vi "HmiScheduler.vi"(7 "Param Screen Title":string, 8 "error in (no error)":errorcluster, 11 "Param Initial VI Path":path) -> (0 "error out":errorcluster)   [LabVIEW 2013]
uses:
  Ctrls/BoutonAPropos.ctl
  Ctrls/BoutonHelp.ctl
  HmiSchedulerAppConfig.ctl
  030 - EVENTS/03 - ToMessageHandlerProcess/ToMessageHandlerEvent.ctl
  030 - EVENTS/03 - ToMessageHandlerProcess/enumMessageCriticity.ctl
  050 - CONFIG/00 - ApplicationConfig/Ctrls/EnumFgvConfigCommand.ctl
  SubVis/enumDeferPanelUpdate.ctl
  030 - EVENTS/EnumFgvEventCommand.ctl
  090 - ERRORS/Ctrls/enumLogAndView.ctl
  040 - SCREENS/enumScreen.ctl
panel:
  out "Logo 600 X 200":picture
  out "ApplicationName":string
  out "ScreenTitle":string
  in  "Simulation":string
  in  "ClearError":bool
  in  "ViewError":bool
  out "LastMessage":string
  out "ProgressBar":u8(slide) scale=0.0..100.0
  out "DateTime":string
  in  "BoutonHelp":T1
  in  "BoutonAPropos":T2
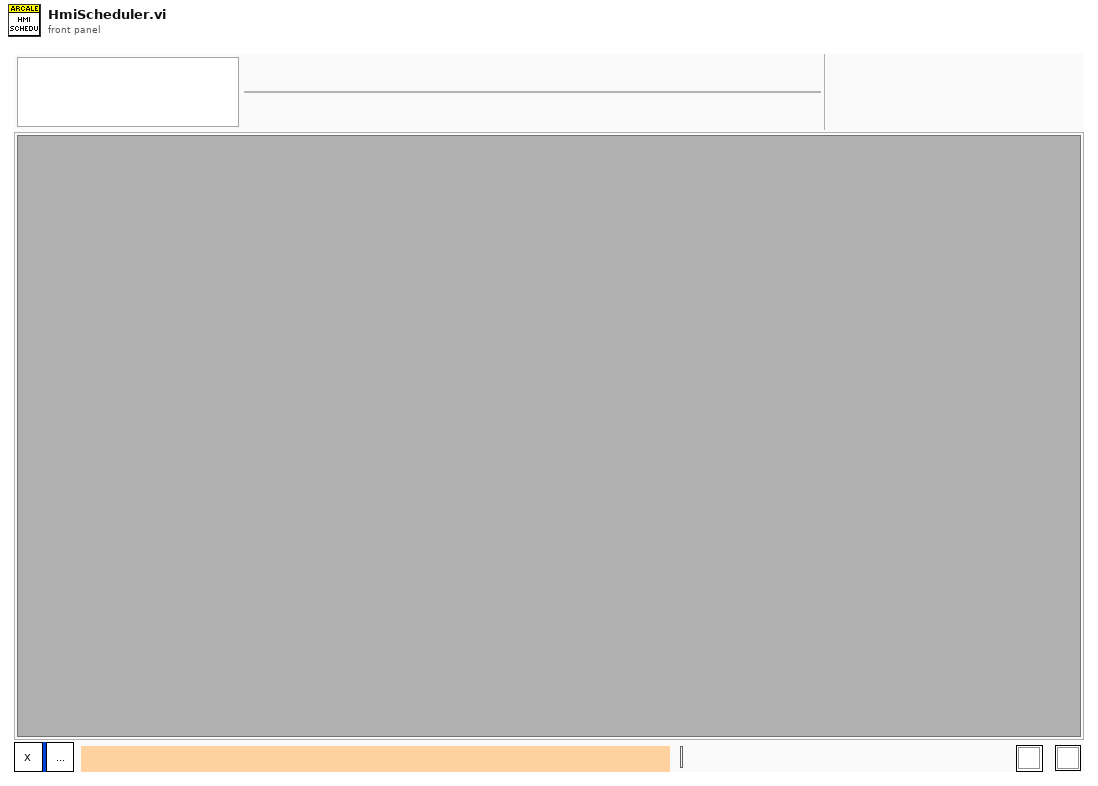
[diagram p1: front panel]
types:
  T1 = typedef "BoutonHelp.ctl" = bool
  T2 = typedef "BoutonAPropos.ctl" = bool
  T3 = typedef "HmiSchedulerAppConfig.ctl" = cluster{"Loaded VI Ref":refnum<vi>, "Loaded Vi Path":path, "AutomaticProgressBarOn":bool, "LastMessage":T4, "Previous loaded VI paths":path[], "Previous loaded Screen title":string[], "Loaded Screen title":string}
  T4 = typedef "ToMessageHandlerEvent.ctl" = cluster{"date / time":timestamp, "Criticity":T5, "Emitter":string, "Message":string}
  T5 = typedef "enumMessageCriticity.ctl" = enum16{"No error", "Info", "Warning", "Error", "Fatal error"}
  T6 = typedef "EnumFgvConfigCommand.ctl" = enum16{"Load", "Get", "Set", "Save To Disk"}
  T7 = enum32{"Invalid", "Standard", "Closed", "Hidden", "Minimized", "Maximized"}
  T8 = typedef "enumDeferPanelUpdate.ctl" = enum16{"suspend layout", "resume layout"}
  T9 = enum8{"Enabled", "Disabled", "Disabled and Grayed Out"}
  T10 = typedef "ApplicationInfos.ctl" = cluster{"ApplicationName":string, "ApplicationVersion":string, "Logo 600X200 path":path, "Logo 400X400 path":path, "Client":string}
  T11 = typedef "ApplicationConfig.ctl" = cluster{"Data Path":path, "MessageHandlerConfig":T12, "Simulation":bool, "Dictionnary":string}
  T12 = typedef "MessageHandlerConfig.ctl" = cluster{"Max log files":u32, "Max messages per file":u32}
  T13 = typedef "EnumFgvEventCommand.ctl" = enum16{"Setup", "Cleanup", "Get"}
  T14 = typedef "enumLogAndView.ctl" = enum16{"Log only", "Log and view"}
  T15 = typedef "enumScreen.ctl" = enum16{"Test screen", "Ecran principal", "LOG", "Setup", "Popup : About", "Popup : View last message", "Popup : WebBrowser help", "Traduction", "Popup : DEBUG Process"}
  T16 = typedef "ToHmiSchedulerCommand.ctl" = enum16{"Load screen", "Lock screen", "Unlock screen", "Close enable", "Close disable", "Start automatic progress bar", "Stop automatic progress bar", "Set progress bar value (0..100)", "Load previous screen", "Close application", "View message", "Clear message", "Set Window State"}
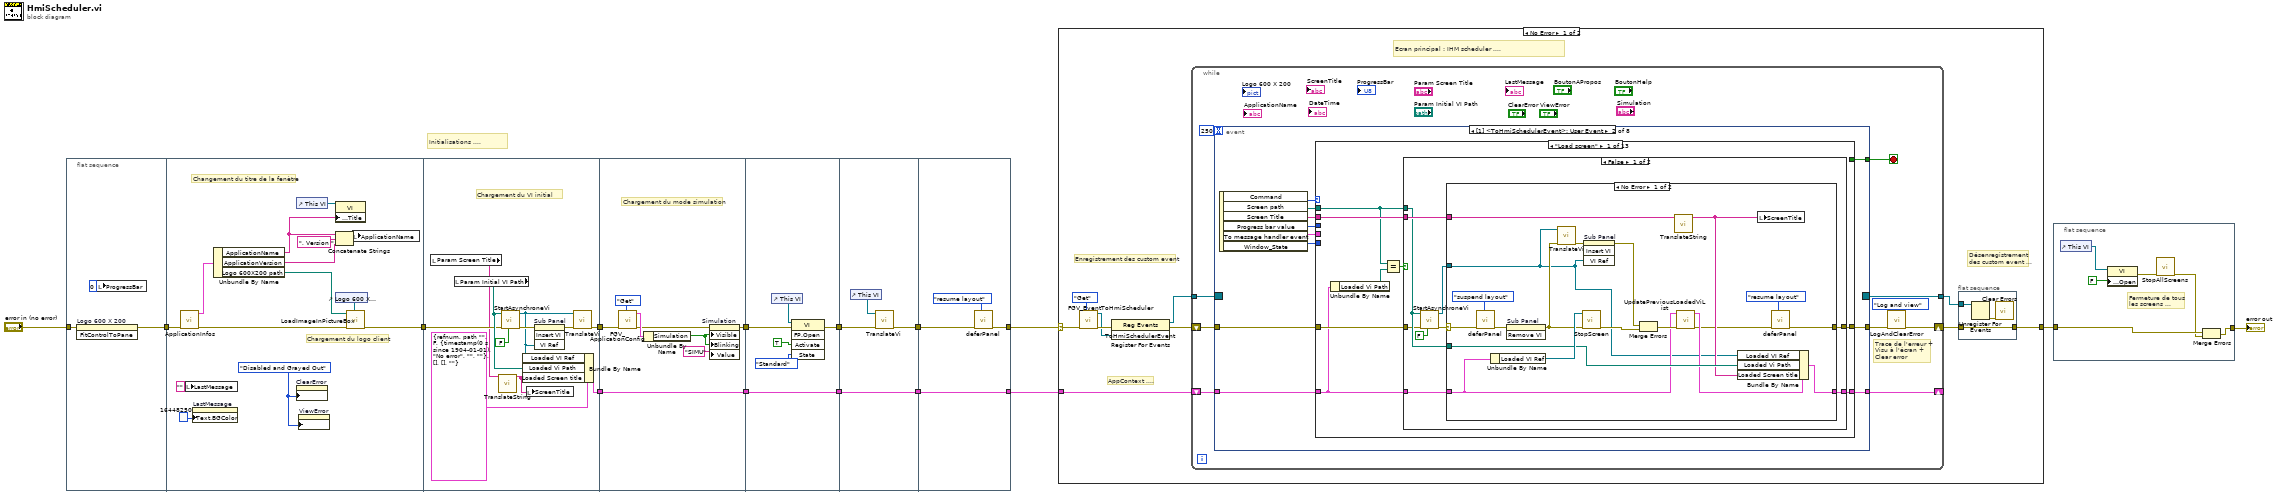
[diagram p0: block diagram]
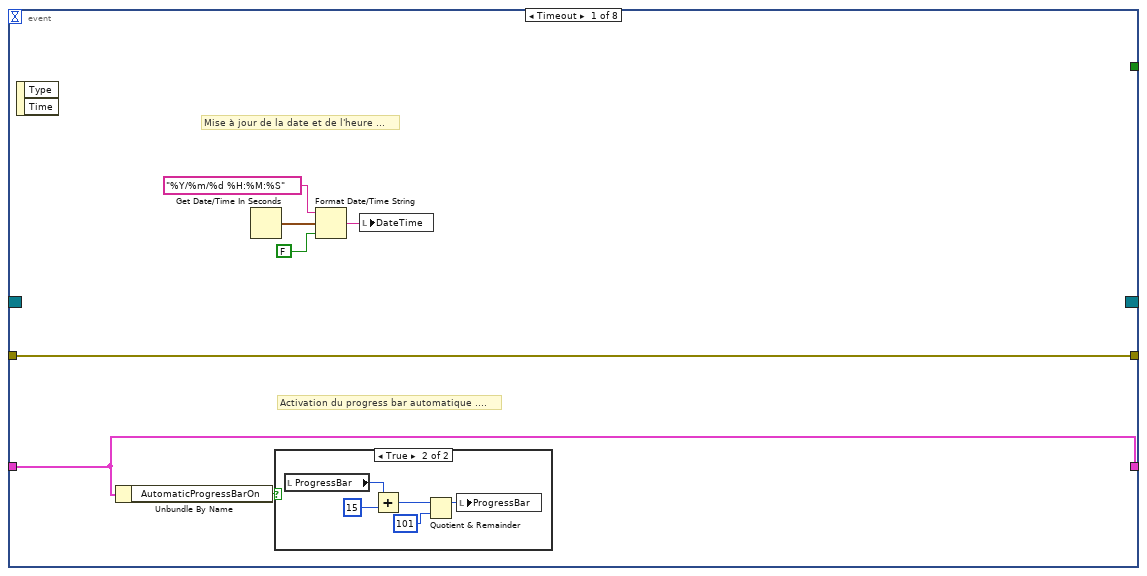
[diagram p2: hidden frame]
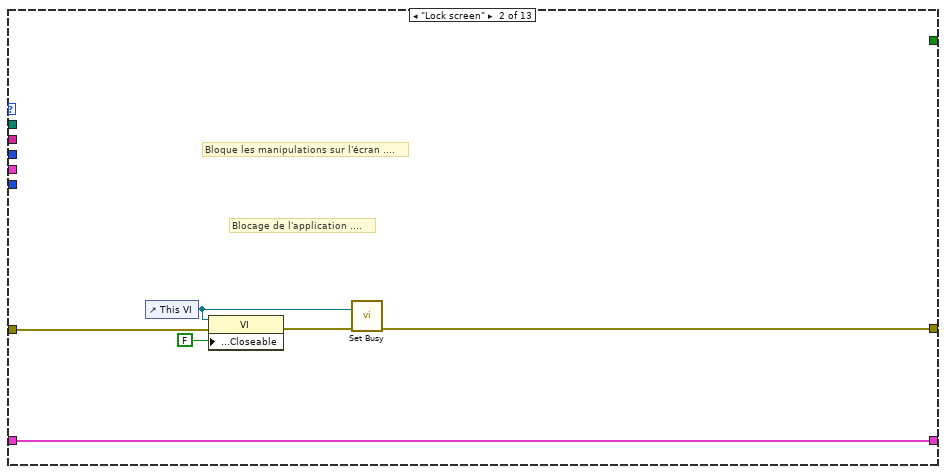
[diagram p6: hidden frame]
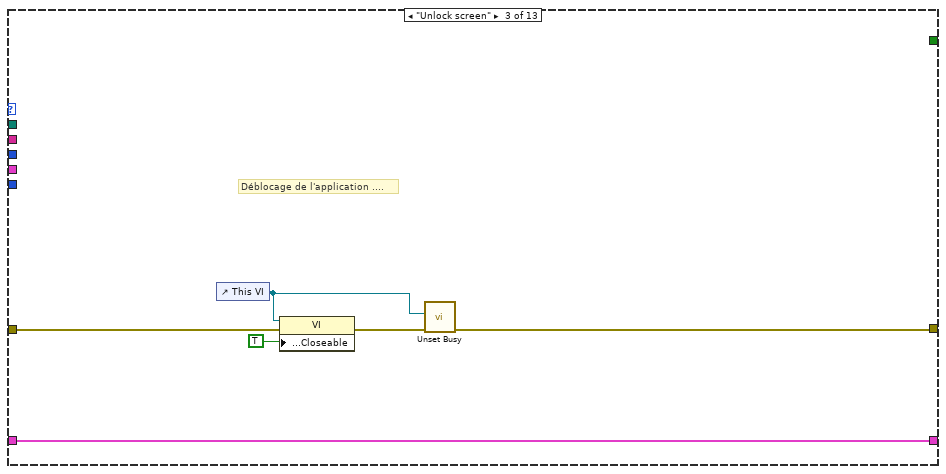
[diagram p7: hidden frame]
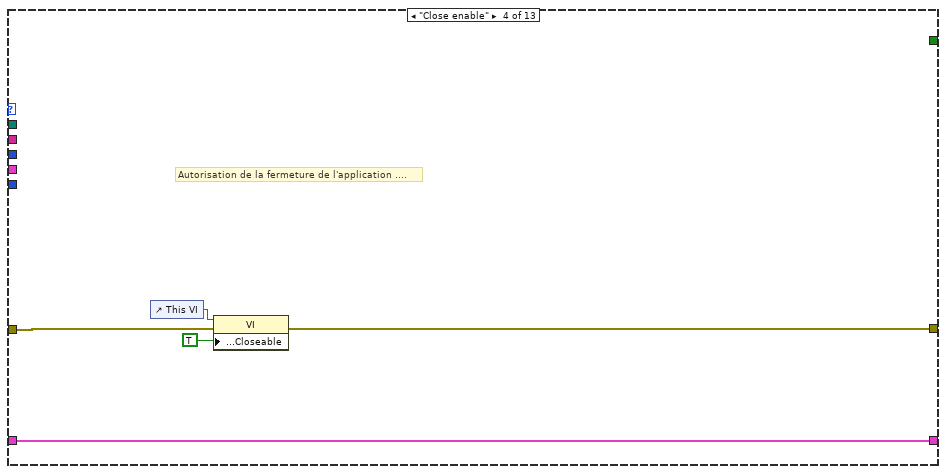
[diagram p8: hidden frame]
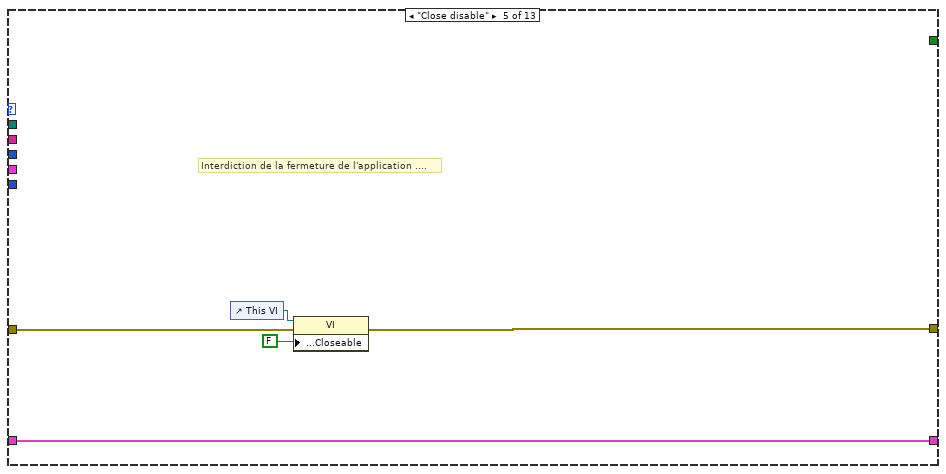
[diagram p9: hidden frame]
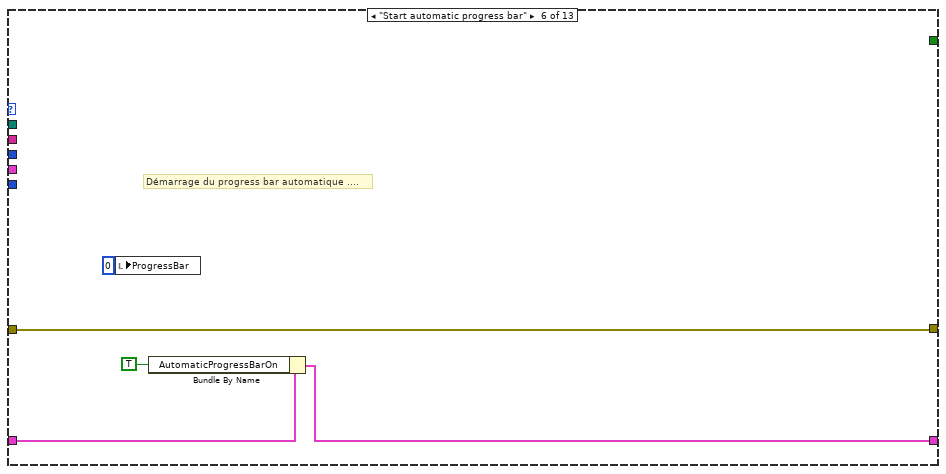
[diagram p10: hidden frame]
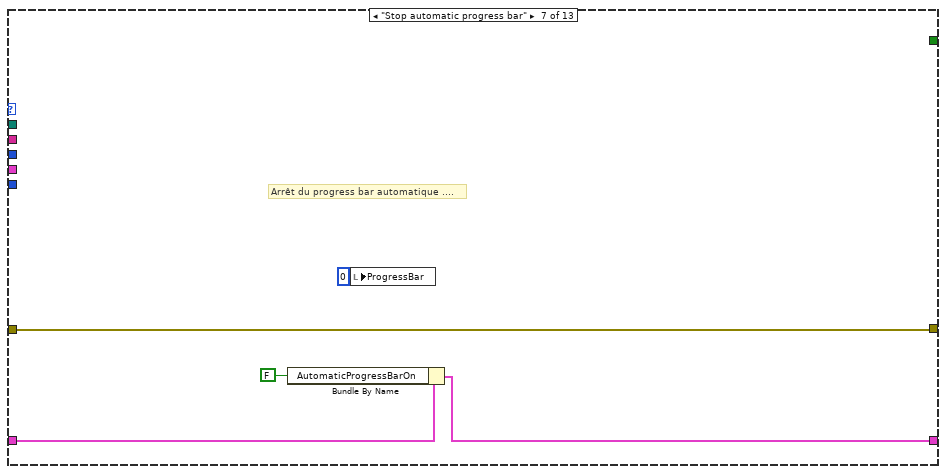
[diagram p11: hidden frame]
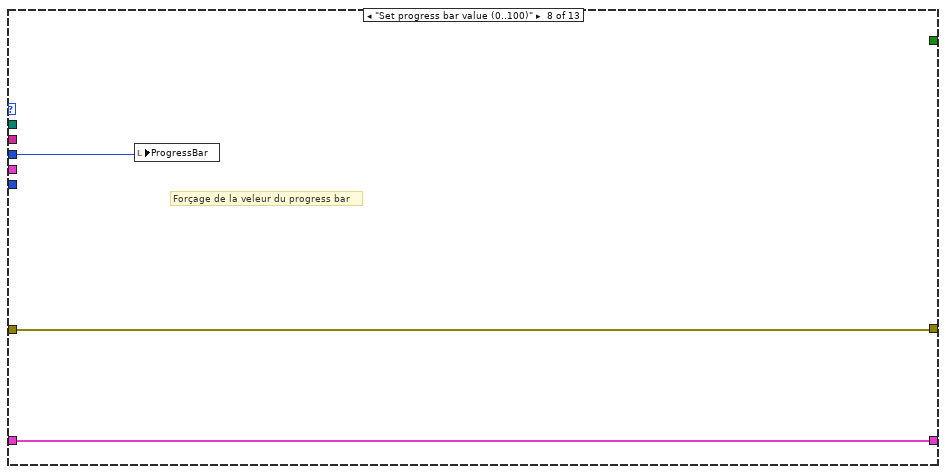
[diagram p12: hidden frame]
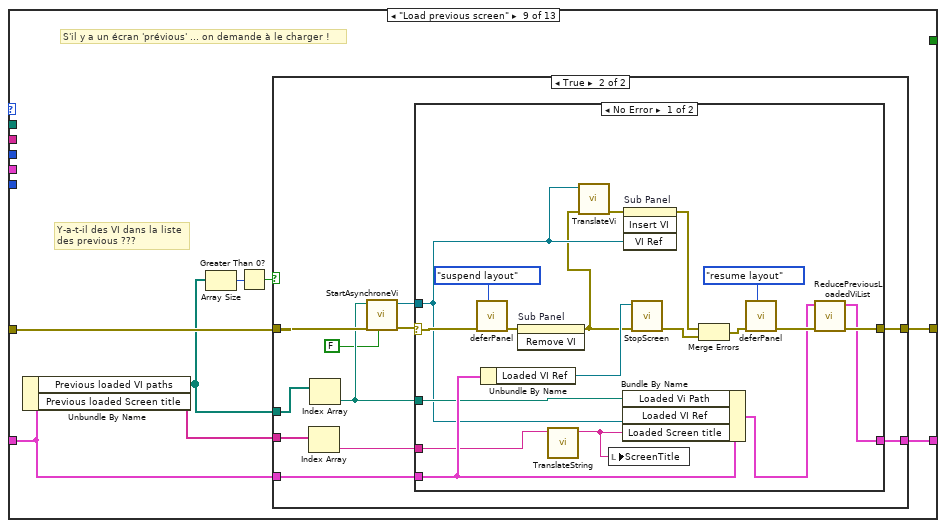
[diagram p13: hidden frame]
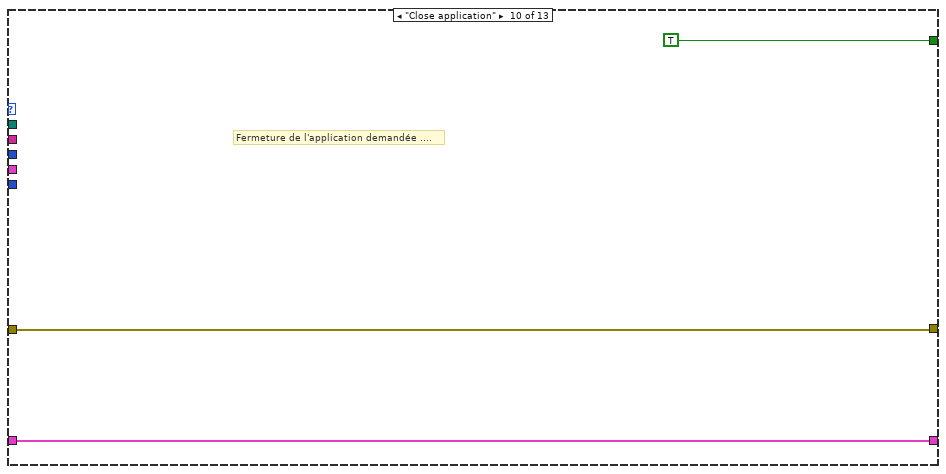
[diagram p16: hidden frame]
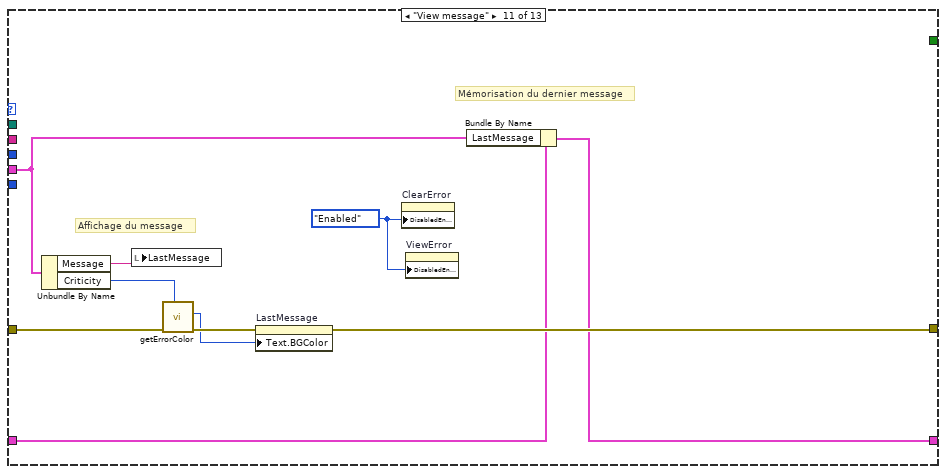
[diagram p17: hidden frame]
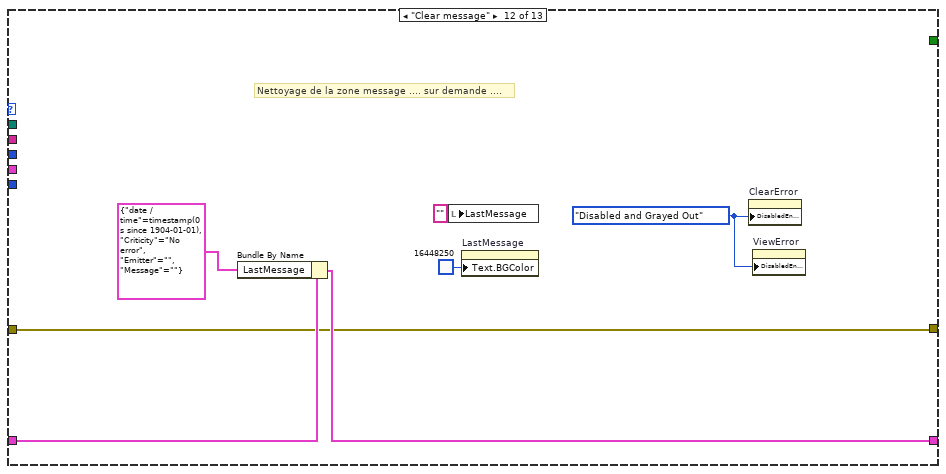
[diagram p18: hidden frame]
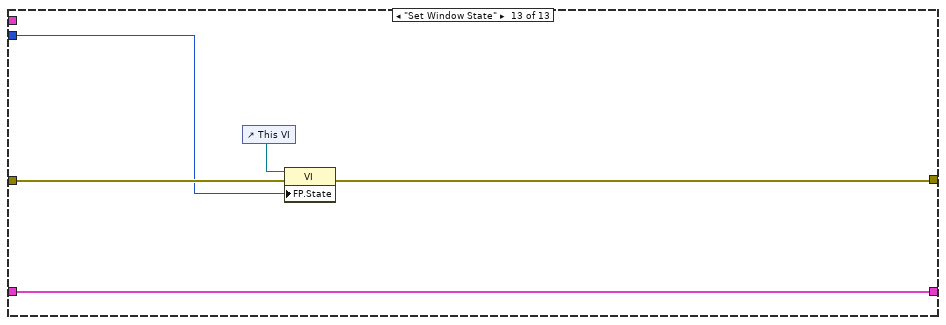
[diagram p19: hidden frame]
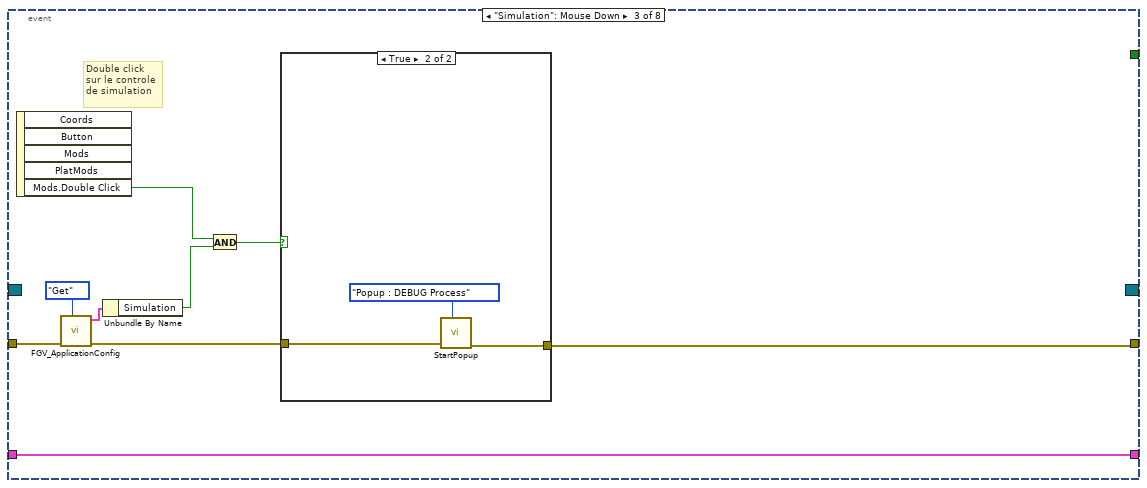
[diagram p20: hidden frame]
diagram:
  # "Initialisations ...."
  n1 = flat-sequence {
    tunnel: "error in (no error)" -> [w18]
    tunnel: [w17] -> w14
    tunnel: w14 -> [w29]
    tunnel: [w30] -> w13
    tunnel: w13 -> [w39]
    tunnel: [w36] -> w10
    tunnel: [w42] -> w9
    tunnel: w10 -> [w50]
    tunnel: w9 -> [w51]
    tunnel: [w46] -> w8
    tunnel: [w51] -> w7
    tunnel: w8 -> [w56]
    tunnel: w7 -> [w57]
    tunnel: [w55] -> w4
    tunnel: [w57] -> w2
    tunnel: w4 -> [w60]
    tunnel: [w59] -> w3
    tunnel: w2 -> [w61]
    tunnel: [w61] -> w1
    tunnel: [w65] -> w12
    tunnel: [w63] -> w11
    tunnel: w3 -> [w64]
    tunnel: w1 -> [w65]
    frame #0 {
      n2 = invoke on="Logo 600 X 200" class="Pict" method="FitControlToPane"(error in=w18) -> (error out=w17:errorcluster)  [unwired: 2 in, 2 out]
      n3 = local write "ProgressBar"(u8 0 ("ProgressBar")) -> ()
    }
    frame #1 {
      w25 = T9."Disabled and Grayed Out" ("Disabled")
      # "Changement du titre de la fenètre"
      # "Chargement du logo client"
      n4 = call "ApplicationInfos.vi"("error in (no error)"=w29) -> ("error out"=w31:errorcluster, "ApplicationInfo"=w24:T10)  [unwired: 9 in]
      n5 = local write "LastMessage"("" ("LastMessage")) -> ()
      n6 = property on="LastMessage" class="Str"("Text.BGColor"=u32 16448250) -> ()  [unwired: 2 in, 2 out]
      n7 = Unbundle By Name(w24) -> ("ApplicationName"=w22:string, "ApplicationVersion"=w20:string, "Logo 600X200 path"=w23:path)
      n8 = property on="ClearError" class="Bool"("DisabledEnum"=w25) -> ()  [unwired: 2 in, 2 out]
      n9 = control-ref of="This VI"() -> (w28:refnum<vi>)
      n10 = property on="ViewError" class="Bool"("DisabledEnum"=w25) -> ()  [unwired: 2 in, 2 out]
      n11 = property class="VI"(reference=w28, "Front Panel.Title"=w22) -> ()  [unwired: 1 in, 2 out]
      n12 = Concatenate Strings(w22, ", Version " ("string"), w20) -> (w21:string)
      n13 = control-ref of="Logo 600 X 200"() -> (w32:refnum<vi>)
      n14 = call "LoadImageInPictureBox.vi"("Pict Refnum In"=w32, "error in (no error)"=w31, "Image file path"=w23) -> ("error out"=w30:errorcluster)  [unwired: 8 in]
      n15 = local write "ApplicationName"(w21) -> ()
    }
    frame #2 {
      # "Chargement du VI initial"
      n16 = local read "Param Screen Title"() -> (w35:string)
      n17 = local read "Param Initial VI Path"() -> (w40:path)
      n18 = call "TranslateString.vi"("String"=w35) -> ("Translated String"=w34:string)  [unwired: 9 in, 1 out]
      n19 = call "StartAsynchroneVi.vi"("Open Front Panel ?"=FALSE, "error in"=w39, "viPathToStart"=w40) -> ("error out"=w41:errorcluster, "vi reference"=w38:refnum<vi>)  [unwired: 7 in]
      n20 = Bundle By Name(cluster=T3 {"Loaded VI Ref"=refnum, "Loaded Vi Path"=path "", "AutomaticProgressBarOn"=FALSE, "LastMessage"={"date / time"=timestamp(0 s since 1904-01-01), "Criticity"=enum."No error", "Emitter"="", "Message"=""}, "Previous loaded VI paths"=[], "Previous loaded Screen title"=[], "Loaded Screen title"=""} ("AppContext"), "Loaded VI Ref"=w38, "Loaded Vi Path"=w40, "Loaded Screen title"=w34) -> (w42:T3)
      n21 = local write "ScreenTitle"(w34) -> ()
      n22 = invoke on="Sub Panel" class="SubPanel" method="Insert VI"(error in=w41, "VI Ref"=w38) -> (error out=w37:errorcluster)  [unwired: 2 in, 3 out]
      n23 = call "TranslateVi.vi"("error in (no error)"=w37, "VI ref"=w38) -> ("error out"=w36:errorcluster)  [unwired: 9 in]
    }
    frame #3 {
      # "Chargement du mode simulation"
      n24 = call "FGV_ApplicationConfig.vi"("Command"=EnumFgvConfigCommand."Get", "error in (no error)"=w50) -> ("error out"=w47:errorcluster, "ApplicationConfigOut"=w48:T11)  [unwired: 8 in]
      n25 = Unbundle By Name(w48) -> ("Simulation"=w45:bool)
      n26 = property on="Simulation" class="Str"(error in=w47, "Visible"=w45, "Blinking"=w45, "Value"="SIMU" ("Simulation")) -> (error out=w46:errorcluster)  [unwired: 1 in, 1 out]
    }
    frame #4 {
      n27 = control-ref of="This VI"() -> (w54:refnum<vi>)
      n28 = invoke class="VI" method="FP.Open"(reference=w54, error in=w56, "Activate"=TRUE ("Activate?"), "State"=T7."Standard") -> (error out=w55:errorcluster)  [unwired: 1 in, 4 out]
    }
    frame #5 {
      n29 = control-ref of="This VI"() -> (w58:refnum<vi>)
      n30 = call "TranslateVi.vi"("error in (no error)"=w60, "VI ref"=w58) -> ("error out"=w59:errorcluster)  [unwired: 9 in]
    }
    frame #6 {
      n31 = call "deferPanel.vi"("EnumDeferPanel"=enumDeferPanelUpdate."resume layout", "errorIn"=w64) -> ("error out"=w63:errorcluster)  [unwired: 9 in]
    }
  }
  n32 = case shown="No Error" w11 {
    selector: w11 -> [w67 w304]
    tunnel: [w66 w304] -> w6
    tunnel: w12 -> [w68 _]
    frame No Error {
      # "Désenregistrement\ndes custom event ..."
      # "Enregistrement des custom event"
      # "AppContext ...."
      # "Ecran principal : IHM scheduler ...."
      n33 = call "FGV_EventToHmiScheduler.vi"("Command"=EnumFgvEventCommand."Get", "error in (no error)"=w67) -> ("error out"=w75:errorcluster, "ToHmiSchedulerEvent"=w72:refnum<user-event>)  [unwired: 8 in]
      n34 = register-events(error in=w75, w72) -> (reference out=w71:refnum<event-registration>, error out=w74:errorcluster)  [unwired: 1 in]
      n35 = while {
        shift-right: [w81] -> w69
        shift-left: w74 -> [w88]
        tunnel: w71 -> [w85]
        tunnel: [w84] -> w70
        shift-right: [w82] -> _
        shift-left: w68 -> [w83]
        stop <- w87 stop-if-true
        # "Trace de l'erreur +\nVisu à l'écran +\nClear error"
        n36 = event shown="[1] <ToHmiSchedulerEvent>: User Event" {
          selector: w85 -> [_ _ _ _ _ _ _ _]
          dyn-events: [_ _ _ _ _ _ _ _] -> w84
          timeout: 250 -> [_ _ _ _ _ _ _ _]
          tunnel: w88 -> [w90 w110 w262 w270 w273 w286 w298 w302]
          tunnel: [w90 w109 w254 w269 w276 w279 w298 w302] -> w80
          tunnel: [_ w103 _ _ _ _ _ TRUE] -> w87
          tunnel: w83 -> [w89 w107 w255 w268 w275 w287 w297 w301]
          tunnel: [w89 w108 w255 w268 w275 w287 w295 w301] -> w82
          event Timeout {
            # "Activation du progress bar automatique ...."
            # "Mise à jour de la date et de l'heure ..."
            n37 = event-data() -> ()  [unwired: 1 in, 2 out]
            n38 = Unbundle By Name(w89) -> ("AutomaticProgressBarOn"=w91:bool)
            n39 = Get Date/Time In Seconds() -> (seconds since 1Jan1904=w95:timestamp)
            n40 = case shown="True" w91 {
              frame False {
              }
              frame True {
                n41 = local read "ProgressBar"() -> (w100:u8)
                n42 = Add(x=w100, y=u8 15) -> (x+y=w98:u8)
                n43 = Quotient & Remainder(x=w98, y=u8 101) -> (x-y*floor(x/y)=w96:u8)  [unwired: 1 out]
                n44 = local write "ProgressBar"(w96) -> ()
              }
            }
            n45 = Format Date/Time String(time format string (%c)="%Y/%m/%d %H:%M:%S", seconds (now)=w95, UTC format=FALSE) -> (date/time string=w92:string)
            n46 = local write "DateTime"(w92) -> ()
          }
          event User Event {
            n47 = event-data() -> ("Command"=w111:T16, "Screen path"=w106:path, "Screen Title"=w104:string, "Progress bar value"=w105:u8, "To message handler event"=w102:T4, "Window_State"=w101:T7)  [unwired: 1 in]
            n48 = case shown="\"Load screen\"" w111 {
              tunnel: w110 -> [w119 w157 w162 w166 w171 w174 w179 w184 w193 w230 w238 w242 w252]
              tunnel: [w118 w153 w159 w165 w170 w174 w179 w184 w192 w230 w240 w242 w251] -> w109
              tunnel: [w117 w155 w161 w164 w169 w175 w180 w186 w188 w229 w234 w243 w250] -> w108
              tunnel: w107 -> [w115 w155 w161 w164 w169 w177 w181 w186 w190 w229 w235 w244 w250]
              tunnel: w106 -> [w112 _ _ _ _ _ _ _ _ _ _ _ _]
              tunnel: w105 -> [_ _ _ _ _ _ _ w185 _ _ _ _ _]
              tunnel: w104 -> [w116 _ _ _ _ _ _ _ _ _ _ _ _]
              tunnel: [_ _ _ _ _ _ _ _ _ TRUE _ _ _] -> w103
              tunnel: w102 -> [_ _ _ _ _ _ _ _ _ _ w233 _ _]
              tunnel: w101 -> [_ _ _ _ _ _ _ _ _ _ _ _ w249]
              frame "Load screen" {
                n49 = Unbundle By Name(w115) -> ("Loaded Vi Path"=w114:path)
                n50 = Equal?(x=w112, y=w114) -> (x = y?=w113:bool)
                n51 = case shown="False" w113 {
                  tunnel: w119 -> [w122 w151]
                  tunnel: [w121 w151] -> w118
                  tunnel: [w126 w150] -> w117
                  tunnel: w116 -> [w125 _]
                  tunnel: w115 -> [w124 w150]
                  tunnel: w112 -> [w123 _]
                  frame False {
                    n52 = call "StartAsynchroneVi.vi"("Open Front Panel ?"=FALSE, "error in"=w122, "viPathToStart"=w123) -> ("error out"=w128:errorcluster, "vi reference"=w127:refnum<vi>)  [unwired: 7 in]
                    n53 = case shown="No Error" w128 {
                      selector: w128 -> [w142 w148]
                      tunnel: [w135 w148] -> w121
                      tunnel: w127 -> [w129 _]
                      tunnel: w124 -> [w138 w149]
                      tunnel: [w136 w149] -> w126
                      tunnel: w123 -> [w144 _]
                      tunnel: w125 -> [w134 _]
                      frame No Error {
                        n54 = call "deferPanel.vi"("EnumDeferPanel"=enumDeferPanelUpdate."suspend layout", "errorIn"=w142) -> ("error out"=w141:errorcluster)  [unwired: 9 in]
                        n55 = Unbundle By Name(w138) -> ("Loaded VI Ref"=w147:refnum<vi>)
                        n56 = invoke on="Sub Panel" class="SubPanel" method="Remove VI"(error in=w141) -> (error out=w131:errorcluster)  [unwired: 2 in, 2 out]
                        n57 = call "TranslateVi.vi"("error in (no error)"=w131, "VI ref"=w129) -> ("error out"=w130:errorcluster)  [unwired: 9 in]
                        n58 = call "StopScreen.vi"("error in (no error)"=w131, "ScreenToStop"=w147) -> ("error out"=w145:errorcluster)  [unwired: 9 in]
                        n59 = invoke on="Sub Panel" class="SubPanel" method="Insert VI"(error in=w130, "VI Ref"=w129) -> (error out=w146:errorcluster)  [unwired: 2 in, 3 out]
                        n60 = Merge Errors(w146, w145) -> (w139:errorcluster)
                        n61 = call "TranslateString.vi"("String"=w134) -> ("Translated String"=w133:string)  [unwired: 9 in, 1 out]
                        n62 = call "UpdatePreviousLoadedViList.vi"("error in (no error)"=w139, "HmiSchedulerAppContextIn"=w138) -> ("error out"=w132:errorcluster, "HmiSchedulerAppContextOut"=w137:T3)  [unwired: 8 in]
                        n63 = Bundle By Name(cluster=w137, "Loaded VI Ref"=w129, "Loaded Vi Path"=w144, "Loaded Screen title"=w133) -> (w136:T3)
                        n64 = local write "ScreenTitle"(w133) -> ()
                        n65 = call "deferPanel.vi"("EnumDeferPanel"=enumDeferPanelUpdate."resume layout", "errorIn"=w132) -> ("error out"=w135:errorcluster)  [unwired: 9 in]
                      }
                      frame Error {
                      }
                    }
                  }
                  frame True {
                    # "On demande de recharger le screen actuellement chargé ... on ne fait rien !!!"
                  }
                }
              }
              frame "Lock screen" {
                # "Blocage de l'application ...."
                # "Bloque les manipulations sur l'écran ...."
                n66 = control-ref of="This VI"() -> (w152:refnum<vi>)
                n67 = property class="VI"(reference=w152, error in=w157, "Front Panel.Closeable"=FALSE ("Front Panel Window:Closeable")) -> (error out=w154:errorcluster)  [unwired: 1 out]
                n68 = call <vilib>:"Set Busy.vi"("error in (no error)"=w154, "VI reference (current VI)"=w152) -> ("error out"=w153:errorcluster)  [unwired: 8 in, 1 out]
              }
              frame "Unlock screen" {
                # "Déblocage de l'application ...."
                n69 = control-ref of="This VI"() -> (w158:refnum<vi>)
                n70 = property class="VI"(reference=w158, error in=w162, "Front Panel.Closeable"=TRUE ("Front Panel Window:Closeable")) -> (error out=w160:errorcluster)  [unwired: 1 out]
                n71 = call <vilib>:"Unset Busy.vi"("error in (no error)"=w160, "VI reference (current VI)"=w158) -> ("error out"=w159:errorcluster)  [unwired: 9 in]
              }
              frame "Close enable" {
                # "Autorisation de la fermeture de l'application ...."
                n72 = control-ref of="This VI"() -> (w168:refnum<vi>)
                n73 = property class="VI"(reference=w168, error in=w166, "Front Panel.Closeable"=TRUE ("Front Panel Window:Closeable")) -> (error out=w165:errorcluster)  [unwired: 1 out]
              }
              frame "Close disable" {
                # "Interdiction de la fermeture de l'application ...."
                n74 = control-ref of="This VI"() -> (w173:refnum<vi>)
                n75 = property class="VI"(reference=w173, error in=w171, "Front Panel.Closeable"=FALSE ("Front Panel Window:Closeable")) -> (error out=w170:errorcluster)  [unwired: 1 out]
              }
              frame "Start automatic progress bar" {
                # "Démarrage du progress bar automatique ...."
                n76 = local write "ProgressBar"(u8 0 ("ProgressBar")) -> ()
                n77 = Bundle By Name(cluster=w177, "AutomaticProgressBarOn"=TRUE) -> (w175:T3)
              }
              frame "Stop automatic progress bar" {
                # "Arrêt du progress bar automatique ...."
                n78 = Bundle By Name(cluster=w181, "AutomaticProgressBarOn"=FALSE) -> (w180:T3)
                n79 = local write "ProgressBar"(u8 0 ("ProgressBar")) -> ()
              }
              frame "Set progress bar value (0..100)" {
                # "Forçage de la veleur du progress bar"
                n80 = local write "ProgressBar"(w185) -> ()
              }
              frame "Load previous screen" {
                # "Y-a-t-il des VI dans la liste\ndes previous ???"
                # "S'il y a un écran 'prévious' ... on demande à le charger !"
                n81 = Unbundle By Name(w190) -> ("Previous loaded VI paths"=w189:path[], "Previous loaded Screen title"=w187:string[])
                n82 = Array Size(array=w189) -> (size(s)=w194:i32)
                n83 = Greater Than 0?(x=w194) -> (x > 0?=w191:bool)
                n84 = case shown="True" w191 {
                  tunnel: w193 -> [w196 w204]
                  tunnel: [w196 w202] -> w192
                  tunnel: w190 -> [w195 w207]
                  tunnel: w189 -> [_ w206]
                  tunnel: [w195 w199] -> w188
                  tunnel: w187 -> [_ w205]
                  frame False {
                    # "Il n'y a pas de prévious screen !"
                  }
                  frame True {
                    n85 = Index Array(array=w205) -> (element=w200:string)  [unwired: 1 in]
                    n86 = Index Array(array=w206) -> (element=w198:path)  [unwired: 1 in]
                    n87 = call "StartAsynchroneVi.vi"("Open Front Panel ?"=FALSE, "error in"=w204, "viPathToStart"=w198) -> ("error out"=w203:errorcluster, "vi reference"=w201:refnum<vi>)  [unwired: 7 in]
                    n88 = case shown="No Error" w203 {
                      selector: w203 -> [w220 w228]
                      tunnel: w207 -> [w219 w227]
                      tunnel: [w216 w228] -> w202
                      tunnel: w201 -> [w212 _]
                      tunnel: w200 -> [w208 _]
                      tunnel: [w214 w227] -> w199
                      tunnel: w198 -> [w213 _]
                      frame No Error {
                        n89 = call "deferPanel.vi"("EnumDeferPanel"=enumDeferPanelUpdate."suspend layout", "errorIn"=w220) -> ("error out"=w223:errorcluster)  [unwired: 9 in]
                        n90 = Unbundle By Name(w219) -> ("Loaded VI Ref"=w218:refnum<vi>)
                        n91 = invoke on="Sub Panel" class="SubPanel" method="Remove VI"(error in=w223) -> (error out=w211:errorcluster)  [unwired: 2 in, 2 out]
                        n92 = call "TranslateString.vi"("String"=w208) -> ("Translated String"=w209:string)  [unwired: 9 in, 1 out]
                        n93 = call "TranslateVi.vi"("error in (no error)"=w211, "VI ref"=w212) -> ("error out"=w210:errorcluster)  [unwired: 9 in]
                        n94 = local write "ScreenTitle"(w209) -> ()
                        n95 = Bundle By Name(cluster=w219, "Loaded Vi Path"=w213, "Loaded VI Ref"=w212, "Loaded Screen title"=w209) -> (w215:T3)
                        n96 = invoke on="Sub Panel" class="SubPanel" method="Insert VI"(error in=w210, "VI Ref"=w212) -> (error out=w226:errorcluster)  [unwired: 2 in, 3 out]
                        n97 = call "StopScreen.vi"("error in (no error)"=w211, "ScreenToStop"=w218) -> ("error out"=w225:errorcluster)  [unwired: 9 in]
                        n98 = Merge Errors(w226, w225) -> (w221:errorcluster)
                        n99 = call "deferPanel.vi"("EnumDeferPanel"=enumDeferPanelUpdate."resume layout", "errorIn"=w221) -> ("error out"=w217:errorcluster)  [unwired: 9 in]
                        n100 = call "ReducePreviousLoadedViList.vi"("error in (no error)"=w217, "HmiSchedulerAppContextIn"=w215) -> ("error out"=w216:errorcluster, "HmiSchedulerAppContextOut"=w214:T3)  [unwired: 8 in]
                      }
                      frame Error {
                      }
                    }
                  }
                }
              }
              frame "Close application" {
                # "Fermeture de l'application demandée ...."
              }
              frame "View message" {
                w232 = T9."Enabled" ("Disabled")
                # "Mémorisation du dernier message"
                # "Affichage du message"
                n101 = Unbundle By Name(w233) -> ("Message"=w241:string, "Criticity"=w239:T5)
                n102 = local write "LastMessage"(w241) -> ()
                n103 = call "getErrorColor.vi"("Criticity"=w239, "error in (no error)"=w238) -> ("error out"=w237:errorcluster, "errorColor"=w236:u32)  [unwired: 8 in]
                n104 = property on="LastMessage" class="Str"(error in=w237, "Text.BGColor"=w236) -> (error out=w240:errorcluster)  [unwired: 1 in, 1 out]
                n105 = property on="ClearError" class="Bool"("DisabledEnum"=w232) -> ()  [unwired: 2 in, 2 out]
                n106 = property on="ViewError" class="Bool"("DisabledEnum"=w232) -> ()  [unwired: 2 in, 2 out]
                n107 = Bundle By Name(cluster=w235, "LastMessage"=w233) -> (w234:T3)
              }
              frame "Clear message" {
                w246 = T9."Disabled and Grayed Out" ("Disabled")
                # "Nettoyage de la zone message .... sur demande ...."
                n108 = Bundle By Name(cluster=w244, "LastMessage"=T4 {"date / time"=timestamp(0 s since 1904-01-01), "Criticity"=enum."No error", "Emitter"="", "Message"=""}) -> (w243:T3)
                n109 = local write "LastMessage"("" ("LastMessage")) -> ()
                n110 = property on="LastMessage" class="Str"("Text.BGColor"=u32 16448250) -> ()  [unwired: 2 in, 2 out]
                n111 = property on="ClearError" class="Bool"("DisabledEnum"=w246) -> ()  [unwired: 2 in, 2 out]
                n112 = property on="ViewError" class="Bool"("DisabledEnum"=w246) -> ()  [unwired: 2 in, 2 out]
              }
              frame "Set Window State" {
                n113 = control-ref of="This VI"() -> (w253:refnum<vi>)
                n114 = property class="VI"(reference=w253, error in=w252, "FP.State"=w249) -> (error out=w251:errorcluster)  [unwired: 1 out]
              }
            }
          }
          event "Simulation": Mouse Down {
            # "Double click\nsur le controle\nde simulation"
            n115 = event-data() -> ("Mods.Double Click"=w258:bool)  [unwired: 1 in, 4 out]
            n116 = call "FGV_ApplicationConfig.vi"("Command"=EnumFgvConfigCommand."Get", "error in (no error)"=w262) -> ("error out"=w261:errorcluster, "ApplicationConfigOut"=w259:T11)  [unwired: 8 in]
            n117 = Unbundle By Name(w259) -> ("Simulation"=w257:bool)
            n118 = And(x=w258, y=w257) -> (x .and. y?=w256:bool)
            n119 = case shown="True" w256 {
              tunnel: w261 -> [w263 w266]
              tunnel: [w263 w264] -> w254
              frame False {
              }
              frame True {
                n120 = call "StartPopup.vi"("Popup"=enumScreen."Popup : DEBUG Process", "error in (no error)"=w266) -> ("error out"=w264:errorcluster)  [unwired: 9 in]
              }
            }
          }
          event Value Change {
            # "Démarrage du popup ABout en détaché !!"
            n121 = event-data() -> ()  [unwired: 1 in, 2 out]
            n122 = call "StartPopup.vi"("Popup"=enumScreen."Popup : About", "error in (no error)"=w270) -> ("error out"=w269:errorcluster)  [unwired: 9 in]
          }
          event "ViewError": Value Change {
            n123 = event-data() -> ()  [unwired: 1 in, 2 out]
            n124 = Unbundle By Name(w275) -> ("LastMessage"=w274:T4)
            n125 = Flatten To String(anything=w274, error in (no error)=w273) -> (data string=w271:string, error out=w272:errorcluster)  [unwired: 2 in, 1 out]
            n126 = call "StartPopup.vi"("Popup"=enumScreen."Popup : View last message", "error in (no error)"=w272, "String parameter"=w271) -> ("error out"=w276:errorcluster)  [unwired: 8 in]
          }
          event Value Change {
            # "On vérifie si un fichier d'aide en ligne existe ?"
            n127 = event-data() -> ()  [unwired: 1 in, 1 out]
            n128 = call "getDataPath.vi"("error in (no error)"=w286) -> ("error out"=w284:errorcluster, "DataPath"=w285:path)  [unwired: 9 in]
            n129 = Build Path(base path=w285, name or relative path="MU.pdf") -> (appended path=w283:path)
            n130 = call <vilib>:"Check if File or Folder Exists.vi"("error in (no error)"=w284, "path"=w283) -> ("error out"=w281:errorcluster, "file or folder exists?"=w282:bool, "dup path"=w280:path)  [unwired: 7 in]
            n131 = case shown="True" w282 {
              tunnel: w281 -> [w288 w293]
              tunnel: w280 -> [_ w292]
              tunnel: [w288 w289] -> w279
              frame False {
                # "Le fichier PDF n'existe pas ... on ne fait rien !"
              }
              frame True {
                # "Le fichier PDF d'aide existe ..."
                n132 = Path To String(path=w292) -> (string=w291:string)
                n133 = call "StartPopup.vi"("Popup"=enumScreen."Popup : WebBrowser help", "error in (no error)"=w293, "String parameter"=w291) -> ("error out"=w289:errorcluster)  [unwired: 8 in]
              }
            }
          }
          event "ClearError": Value Change {
            w294 = T9."Disabled and Grayed Out" ("Disabled")
            # "Nettoyage de l'erreur courante ...."
            n134 = event-data() -> ()  [unwired: 1 in, 2 out]
            n135 = local write "LastMessage"("" ("LastMessage")) -> ()
            n136 = property on="LastMessage" class="Str"("Text.BGColor"=u32 16448250) -> ()  [unwired: 2 in, 2 out]
            n137 = Bundle By Name(cluster=w297, "LastMessage"=T4 {"date / time"=timestamp(0 s since 1904-01-01), "Criticity"=enum."No error", "Emitter"="", "Message"=""}) -> (w295:T3)
            n138 = property on="ClearError" class="Bool"("DisabledEnum"=w294) -> ()  [unwired: 2 in, 2 out]
            n139 = property on="ViewError" class="Bool"("DisabledEnum"=w294) -> ()  [unwired: 2 in, 2 out]
          }
          event Panel Close {
            # "Fermeture du panel courant ...."
            n140 = event-data() -> ()  [unwired: 1 in, 3 out]
          }
        }
        n141 = call "LogAndClearError.vi"("Log and view ?"=enumLogAndView."Log and view", "error in (no error)"=w80) -> ("error out"=w81:errorcluster)  [unwired: 9 in]
      }
      n142 = flat-sequence {
        tunnel: w70 -> [w78]
        tunnel: w69 -> [w76]
        tunnel: [w76] -> w66
        frame #0 {
          n143 = Unregister For Events(event registration refnum=w78) -> (error out=w77:errorcluster)  [unwired: 1 in]
          n144 = call <vilib>:"Clear Errors.vi"("error in (no error)"=w77) -> ()  [unwired: 6 in, 1 out]
        }
      }
    }
    frame Error {
    }
  }
  n145 = flat-sequence {
    tunnel: w6 -> [w307]
    tunnel: [w306] -> w5
    frame #0 {
      # "Fermeture de tous\nles screens ..."
      n146 = control-ref of="This VI"() -> (w309:refnum<vi>)
      n147 = property class="VI"(reference=w309, "Front Panel.Open"=FALSE ("Front Panel Window:Open")) -> (error out=w308:errorcluster)  [unwired: 1 in, 1 out]
      n148 = call "StopAllScreens.vi"("error in (no error)"=w308) -> ("error out"=w305:errorcluster)  [unwired: 10 in]
      n149 = Merge Errors(w307, w305) -> (w306:errorcluster)
    }
  }
  "error out" <- w5
